vi "Tray_Search_ArrTrueIndex.vi"(6 "SearchStatus":bool=TRUE, 7 "Direction":u16=7, 10 "index":i32, 11 "Input_Arr":bool[][](array[boolean])) -> (1 "Status":bool, 2 "SearchTrueIndex":i32, 3 "indexTransXY":cluster{"Y":i32, "X":i32})   [LabVIEW 2015]
panel:
  out "indexTrans":i32
  out "Out XY 2":cluster{"Y":i32, "X":i32}
  out "Out XY":cluster{"Y":i32, "X":i32}
  out "Out PutArr":bool[][](array[boolean])
  # "X=(8-Y)-1\nY=(21-X)-1"
  # "4 6"
  # "8*21"
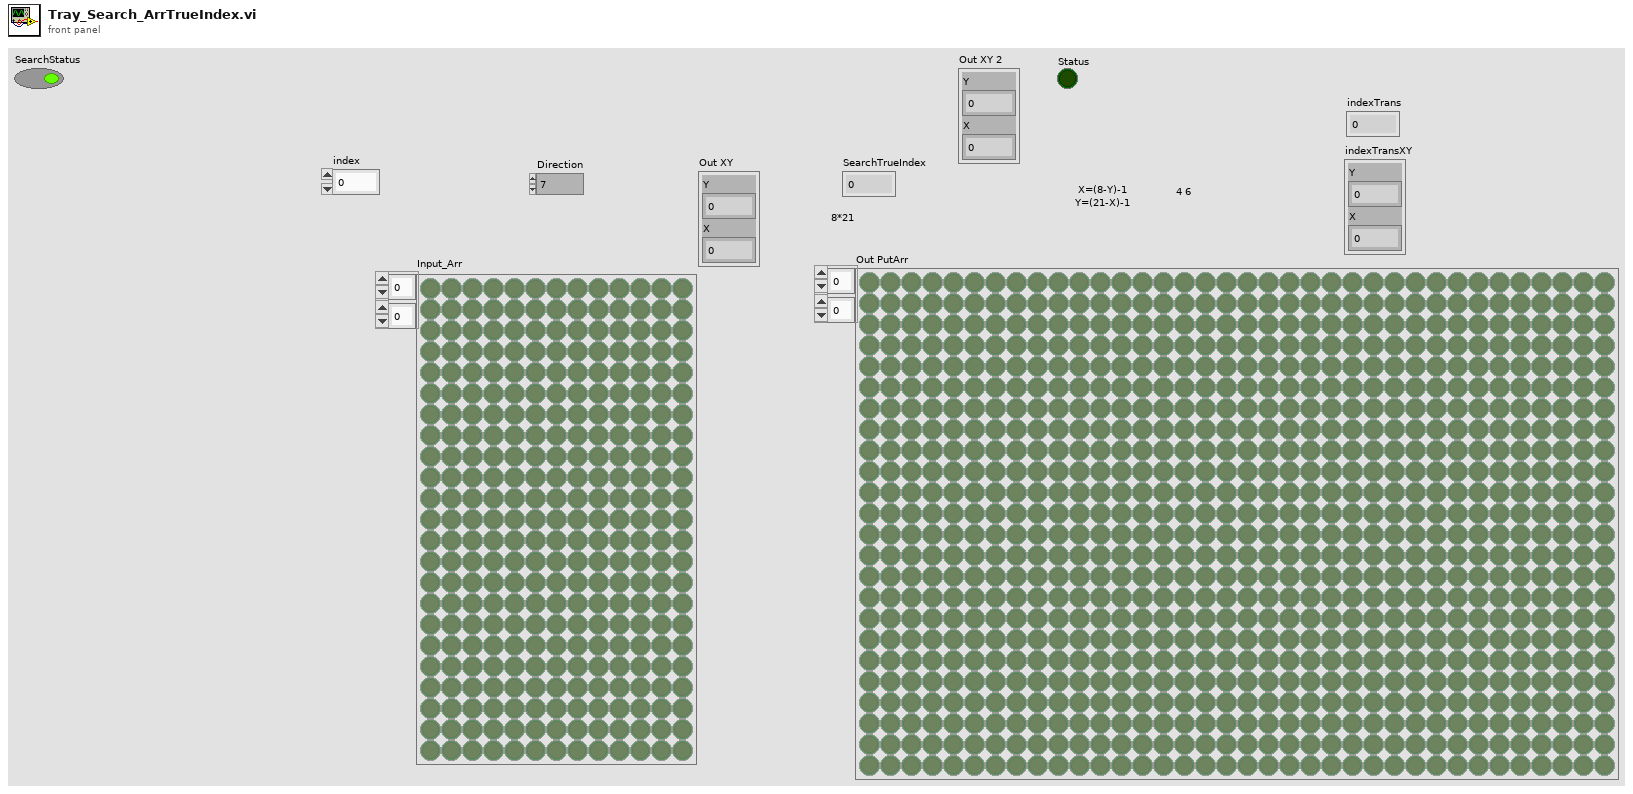
[diagram p1: front panel]
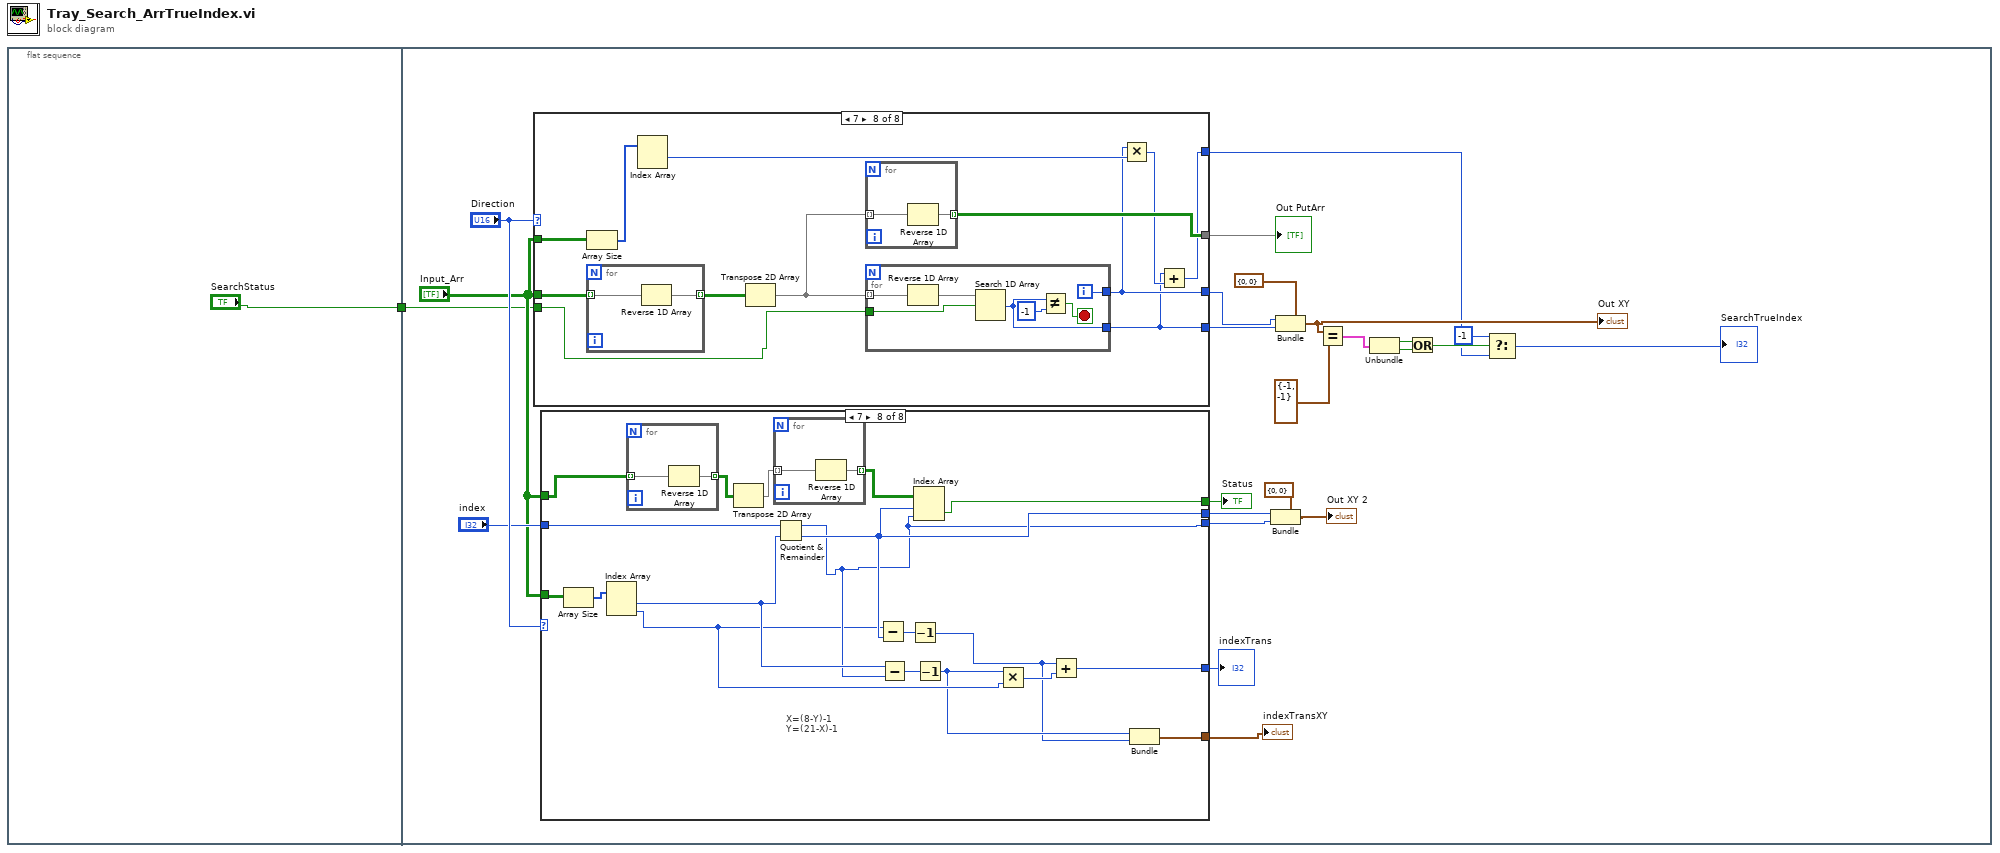
[diagram p0: block diagram]
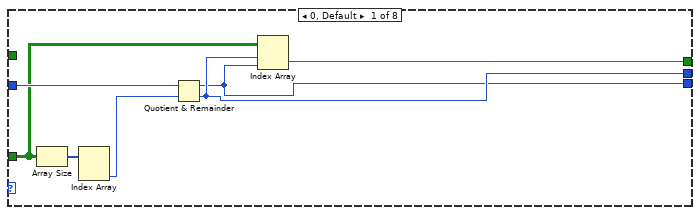
[diagram p2: hidden frame]
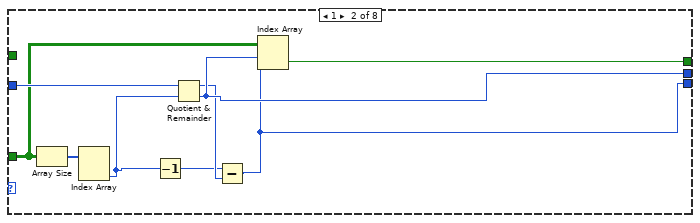
[diagram p3: hidden frame]
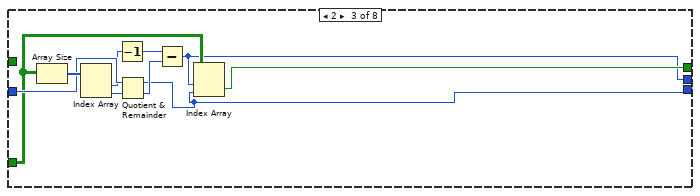
[diagram p4: hidden frame]
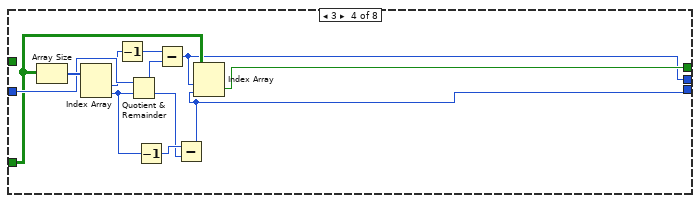
[diagram p5: hidden frame]
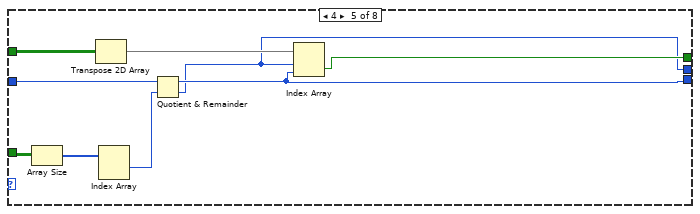
[diagram p6: hidden frame]
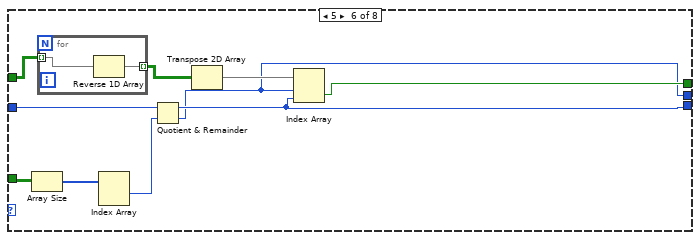
[diagram p7: hidden frame]
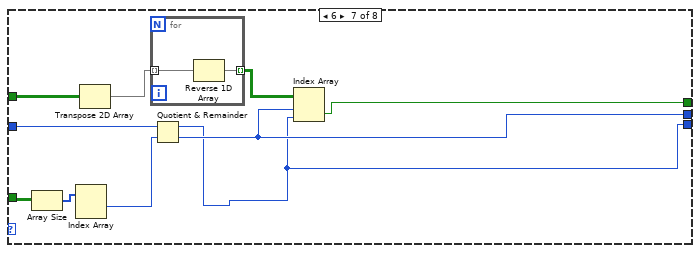
[diagram p8: hidden frame]
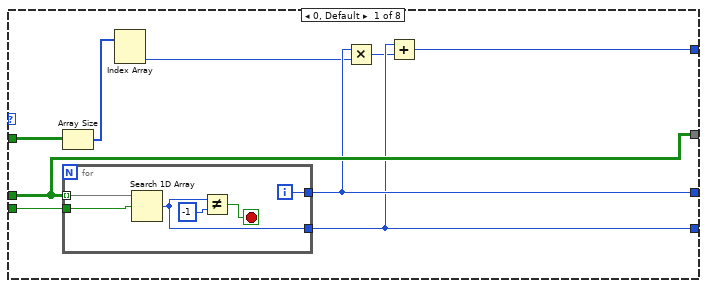
[diagram p9: hidden frame]
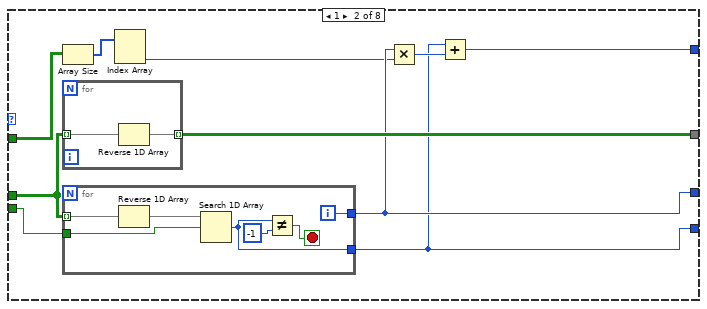
[diagram p10: hidden frame]
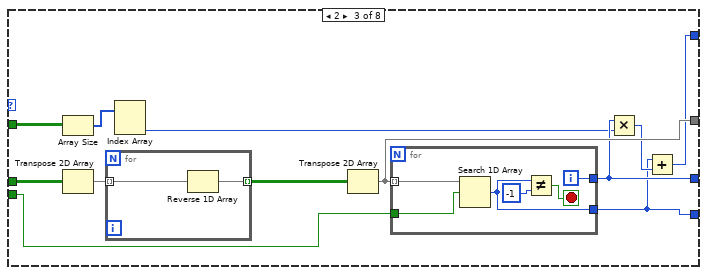
[diagram p11: hidden frame]
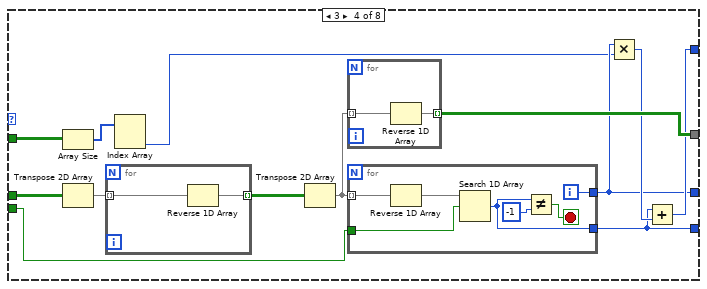
[diagram p12: hidden frame]
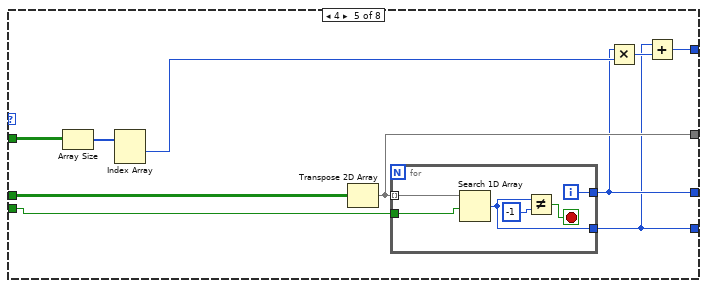
[diagram p13: hidden frame]
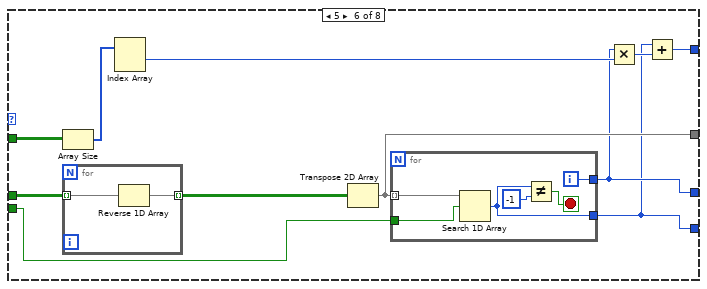
[diagram p14: hidden frame]
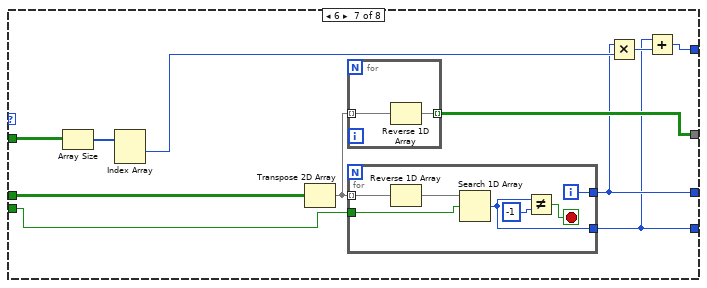
[diagram p15: hidden frame]
diagram:
  n1 = flat-sequence {
    tunnel: ["SearchStatus"] -> w1
    tunnel: w1 -> [w3]
    frame #0 {
    }
    frame #1 {
      n2 = case shown="7" "Direction" {
        tunnel: "Input_Arr" -> [w128 w144 w165 w186 w207 w224 w241 w262]
        tunnel: [w125 w139 w158 w177 w201 w217 w236 w256] -> w25
        tunnel: [w124 w138 w157 w176 w200 w216 w235 w255] -> w24
        tunnel: [w128 w143 w162 w182 w206 w222 w242 w263] -> w23
        tunnel: "Input_Arr" -> [w127 w140 w159 w179 w202 w218 w237 w257]
        tunnel: [w122 w137 w156 w178 w199 w215 w234 w254] -> w16
        tunnel: w3 -> [w120 w135 w154 w174 w198 w214 w233 w253]
        frame 0, Default {
          n3 = Array Size(array=w127) -> (size(s)=w126:i32[])
          n4 = for {
            tunnel: w128 -> [w134] mode=indexing
            tunnel: [w131] -> w125
            tunnel: [w130] -> w124
            tunnel: w120 -> [w129]
            i -> [w131]
            stop <- w132 stop-if-true
            n5 = Search 1D Array(1D array=w134, element=w129) -> (index of element=w130:i32)  [unwired: 1 in]
            n6 = Not Equal?(x=w130, y=-1) -> (x != y?=w132:bool)
          }
          n7 = Index Array(array=w126) -> (element #2=w121:i32)  [unwired: 2 in, 1 out]
          n8 = Multiply(x=w125, y=w121) -> (x*y=w123:i32)
          n9 = Add(x=w124, y=w123) -> (x+y=w122:i32)
        }
        frame 1 {
          n10 = Array Size(array=w140) -> (size(s)=w142:i32[])
          n11 = for {
            tunnel: w144 -> [w146] mode=indexing
            tunnel: [w145] -> w143 mode=indexing
            n12 = Reverse 1D Array(array=w146) -> (reversed array=w145:bool[])
          }
          n13 = for {
            tunnel: w144 -> [w153] mode=indexing
            tunnel: [w150] -> w139
            tunnel: [w149] -> w138
            tunnel: w135 -> [w147]
            i -> [w150]
            stop <- w151 stop-if-true
            n14 = Reverse 1D Array(array=w153) -> (reversed array=w148:bool[])
            n15 = Search 1D Array(1D array=w148, element=w147) -> (index of element=w149:i32)  [unwired: 1 in]
            n16 = Not Equal?(x=w149, y=-1) -> (x != y?=w151:bool)
          }
          n17 = Index Array(array=w142) -> (element #2=w136:i32)  [unwired: 2 in, 1 out]
          n18 = Multiply(x=w139, y=w136) -> (x*y=w141:i32)
          n19 = Add(x=w138, y=w141) -> (x+y=w137:i32)
        }
        frame 2 {
          n20 = Array Size(array=w159) -> (size(s)=w161:i32[])
          n21 = Transpose 2D Array(2D array=w165) -> (transposed array=w164:bool[][])
          n22 = for {
            tunnel: w164 -> [w167] mode=indexing
            tunnel: [w166] -> w163 mode=indexing
            n23 = Reverse 1D Array(array=w167) -> (reversed array=w166:bool[])
          }
          n24 = Index Array(array=w161) -> (element #2=w155:i32)  [unwired: 2 in, 1 out]
          n25 = Transpose 2D Array(2D array=w163) -> (transposed array=w162:bool[][])
          n26 = for {
            tunnel: w162 -> [w169] mode=indexing
            tunnel: [w171] -> w158
            tunnel: [w170] -> w157
            tunnel: w154 -> [w168]
            i -> [w171]
            stop <- w172 stop-if-true
            n27 = Search 1D Array(1D array=w169, element=w168) -> (index of element=w170:i32)  [unwired: 1 in]
            n28 = Not Equal?(x=w170, y=-1) -> (x != y?=w172:bool)
          }
          n29 = Multiply(x=w158, y=w155) -> (x*y=w160:i32)
          n30 = Add(x=w157, y=w160) -> (x+y=w156:i32)
        }
        frame 3 {
          n31 = Array Size(array=w179) -> (size(s)=w181:i32[])
          n32 = Transpose 2D Array(2D array=w186) -> (transposed array=w185:bool[][])
          n33 = for {
            tunnel: w185 -> [w190] mode=indexing
            tunnel: [w189] -> w184 mode=indexing
            n34 = Reverse 1D Array(array=w190) -> (reversed array=w189:bool[])
          }
          n35 = Index Array(array=w181) -> (element #2=w175:i32)  [unwired: 2 in, 1 out]
          n36 = Transpose 2D Array(2D array=w184) -> (transposed array=w183:bool[][])
          n37 = for {
            tunnel: w183 -> [w188] mode=indexing
            tunnel: [w187] -> w182 mode=indexing
            n38 = Reverse 1D Array(array=w188) -> (reversed array=w187:bool[])
          }
          n39 = for {
            tunnel: w183 -> [w193] mode=indexing
            tunnel: [w195] -> w177
            tunnel: [w194] -> w176
            tunnel: w174 -> [w191]
            i -> [w195]
            stop <- w196 stop-if-true
            n40 = Reverse 1D Array(array=w193) -> (reversed array=w192:bool[])
            n41 = Search 1D Array(1D array=w192, element=w191) -> (index of element=w194:i32)  [unwired: 1 in]
            n42 = Not Equal?(x=w194, y=-1) -> (x != y?=w196:bool)
          }
          n43 = Multiply(x=w177, y=w175) -> (x*y=w180:i32)
          n44 = Add(x=w176, y=w180) -> (x+y=w178:i32)
        }
        frame 4 {
          n45 = Array Size(array=w202) -> (size(s)=w205:i32[])
          n46 = Index Array(array=w205) -> (element #1=w204:i32)  [unwired: 2 in, 1 out]
          n47 = Transpose 2D Array(2D array=w207) -> (transposed array=w206:bool[][])
          n48 = for {
            tunnel: w206 -> [w211] mode=indexing
            tunnel: [w209] -> w200
            tunnel: [w210] -> w201
            tunnel: w198 -> [w208]
            i -> [w210]
            stop <- w212 stop-if-true
            n49 = Search 1D Array(1D array=w211, element=w208) -> (index of element=w209:i32)  [unwired: 1 in]
            n50 = Not Equal?(x=w209, y=-1) -> (x != y?=w212:bool)
          }
          n51 = Multiply(x=w201, y=w204) -> (x*y=w203:i32)
          n52 = Add(x=w200, y=w203) -> (x+y=w199:i32)
        }
        frame 5 {
          n53 = Array Size(array=w218) -> (size(s)=w221:i32[])
          n54 = for {
            tunnel: w224 -> [w226] mode=indexing
            tunnel: [w225] -> w223 mode=indexing
            n55 = Reverse 1D Array(array=w226) -> (reversed array=w225:bool[])
          }
          n56 = Index Array(array=w221) -> (element #1=w220:i32)  [unwired: 2 in, 1 out]
          n57 = Transpose 2D Array(2D array=w223) -> (transposed array=w222:bool[][])
          n58 = for {
            tunnel: w222 -> [w230] mode=indexing
            tunnel: [w229] -> w216
            tunnel: [w228] -> w217
            tunnel: w214 -> [w227]
            i -> [w228]
            stop <- w231 stop-if-true
            n59 = Search 1D Array(1D array=w230, element=w227) -> (index of element=w229:i32)  [unwired: 1 in]
            n60 = Not Equal?(x=w229, y=-1) -> (x != y?=w231:bool)
          }
          n61 = Multiply(x=w217, y=w220) -> (x*y=w219:i32)
          n62 = Add(x=w216, y=w219) -> (x+y=w215:i32)
        }
        frame 6 {
          n63 = Array Size(array=w237) -> (size(s)=w240:i32[])
          n64 = Index Array(array=w240) -> (element #1=w239:i32)  [unwired: 2 in, 1 out]
          n65 = Transpose 2D Array(2D array=w241) -> (transposed array=w243:bool[][])
          n66 = for {
            tunnel: w243 -> [w245] mode=indexing
            tunnel: [w244] -> w242 mode=indexing
            n67 = Reverse 1D Array(array=w245) -> (reversed array=w244:bool[])
          }
          n68 = for {
            tunnel: w243 -> [w250] mode=indexing
            tunnel: [w247] -> w235
            tunnel: [w248] -> w236
            tunnel: w233 -> [w246]
            i -> [w248]
            stop <- w251 stop-if-true
            n69 = Reverse 1D Array(array=w250) -> (reversed array=w249:bool[])
            n70 = Search 1D Array(1D array=w249, element=w246) -> (index of element=w247:i32)  [unwired: 1 in]
            n71 = Not Equal?(x=w247, y=-1) -> (x != y?=w251:bool)
          }
          n72 = Multiply(x=w236, y=w239) -> (x*y=w238:i32)
          n73 = Add(x=w235, y=w238) -> (x+y=w234:i32)
        }
        frame 7 {
          n74 = Array Size(array=w257) -> (size(s)=w260:i32[])
          n75 = for {
            tunnel: w262 -> [w266] mode=indexing
            tunnel: [w265] -> w261 mode=indexing
            n76 = Reverse 1D Array(array=w266) -> (reversed array=w265:bool[])
          }
          n77 = Index Array(array=w260) -> (element #1=w259:i32)  [unwired: 2 in, 1 out]
          n78 = Transpose 2D Array(2D array=w261) -> (transposed array=w264:bool[][])
          n79 = for {
            tunnel: w264 -> [w268] mode=indexing
            tunnel: [w267] -> w263 mode=indexing
            n80 = Reverse 1D Array(array=w268) -> (reversed array=w267:bool[])
          }
          n81 = for {
            tunnel: w264 -> [w273] mode=indexing
            tunnel: [w270] -> w255
            tunnel: [w271] -> w256
            tunnel: w253 -> [w269]
            i -> [w271]
            stop <- w274 stop-if-true
            n82 = Reverse 1D Array(array=w273) -> (reversed array=w272:bool[])
            n83 = Search 1D Array(1D array=w272, element=w269) -> (index of element=w270:i32)  [unwired: 1 in]
            n84 = Not Equal?(x=w270, y=-1) -> (x != y?=w274:bool)
          }
          n85 = Multiply(x=w256, y=w259) -> (x*y=w258:i32)
          n86 = Add(x=w255, y=w258) -> (x+y=w254:i32)
        }
      }
      "Out PutArr" <- w23
      n87 = case shown="7" "Direction" {
        tunnel: "index" -> [w32 w41 w51 w62 w70 w80 w92 w113]
        tunnel: "Input_Arr" -> [w30 w40 w50 w61 w71 w81 w93 w114]
        tunnel: [w29 w39 w46 w59 w64 w75 w90 w107] -> w10
        tunnel: [w28 w35 w43 w53 w65 w76 w85 w104] -> w9
        tunnel: [w27 w38 w49 w60 w68 w78 w91 w112] -> w8
        tunnel: "Input_Arr" -> [_ _ _ _ w67 w74 w89 w109]
        tunnel: [_ _ _ _ _ _ _ w100] -> w5
        tunnel: [_ _ _ _ _ _ _ w97] -> w4
        frame 0, Default {
          n88 = Array Size(array=w30) -> (size(s)=w33:i32[])
          n89 = Index Array(array=w33) -> (element #2=w31:i32)  [unwired: 2 in, 1 out]
          n90 = Quotient & Remainder(x=w32, y=w31) -> (x-y*floor(x/y)=w28:i32, floor(x/y)=w29:i32)
          n91 = Index Array(array=w30, index (row)=w29, index (col)=w28) -> (element=w27:bool)
        }
        frame 1 {
          n92 = Array Size(array=w40) -> (size(s)=w42:i32[])
          n93 = Index Array(array=w42) -> (element #2=w36:i32)  [unwired: 2 in, 1 out]
          n94 = Decrement(x=w36) -> (x-1=w34:i32)
          n95 = Quotient & Remainder(x=w41, y=w36) -> (x-y*floor(x/y)=w37:i32, floor(x/y)=w39:i32)
          n96 = Subtract(x=w34, y=w37) -> (x-y=w35:i32)
          n97 = Index Array(array=w40, index (row)=w39, index (col)=w35) -> (element=w38:bool)
        }
        frame 2 {
          n98 = Array Size(array=w50) -> (size(s)=w52:i32[])
          n99 = Index Array(array=w52) -> (element #1=w44:i32, element #2=w48:i32)  [unwired: 2 in]
          n100 = Decrement(x=w44) -> (x-1=w45:i32)
          n101 = Quotient & Remainder(x=w51, y=w48) -> (x-y*floor(x/y)=w43:i32, floor(x/y)=w47:i32)
          n102 = Subtract(x=w45, y=w47) -> (x-y=w46:i32)
          n103 = Index Array(array=w50, index (row)=w46, index (col)=w43) -> (element=w49:bool)
        }
        frame 3 {
          n104 = Array Size(array=w61) -> (size(s)=w63:i32[])
          n105 = Index Array(array=w63) -> (element #1=w57:i32, element #2=w56:i32)  [unwired: 2 in]
          n106 = Decrement(x=w57) -> (x-1=w58:i32)
          n107 = Quotient & Remainder(x=w62, y=w56) -> (floor(x/y)=w54:i32)  [unwired: 1 out]
          n108 = Decrement(x=w56) -> (x-1=w55:i32)
          n109 = Subtract(x=w58, y=w54) -> (x-y=w59:i32)
          n110 = Subtract(x=w55, y=w54) -> (x-y=w53:i32)
          n111 = Index Array(array=w61, index (row)=w59, index (col)=w53) -> (element=w60:bool)
        }
        frame 4 {
          n112 = Array Size(array=w71) -> (size(s)=w72:i32[])
          n113 = Transpose 2D Array(2D array=w67) -> (transposed array=w66:bool[][])
          n114 = Index Array(array=w72) -> (element #1=w69:i32)  [unwired: 2 in, 1 out]
          n115 = Quotient & Remainder(x=w70, y=w69) -> (x-y*floor(x/y)=w65:i32, floor(x/y)=w64:i32)
          n116 = Index Array(array=w66, index (row)=w64, index (col)=w65) -> (element=w68:bool)
        }
        frame 5 {
          n117 = Array Size(array=w81) -> (size(s)=w82:i32[])
          n118 = for {
            tunnel: [w84] -> w73 mode=indexing
            tunnel: w74 -> [w83] mode=indexing
            n119 = Reverse 1D Array(array=w83) -> (reversed array=w84:bool[])
          }
          n120 = Index Array(array=w82) -> (element #1=w79:i32)  [unwired: 2 in, 1 out]
          n121 = Quotient & Remainder(x=w80, y=w79) -> (x-y*floor(x/y)=w76:i32, floor(x/y)=w75:i32)
          n122 = Transpose 2D Array(2D array=w73) -> (transposed array=w77:bool[][])
          n123 = Index Array(array=w77, index (row)=w75, index (col)=w76) -> (element=w78:bool)
        }
        frame 6 {
          n124 = Array Size(array=w93) -> (size(s)=w94:i32[])
          n125 = Index Array(array=w94) -> (element #1=w86:i32)  [unwired: 2 in, 1 out]
          n126 = Transpose 2D Array(2D array=w89) -> (transposed array=w88:bool[][])
          n127 = for {
            tunnel: w88 -> [w96] mode=indexing
            tunnel: [w95] -> w87 mode=indexing
            n128 = Reverse 1D Array(array=w96) -> (reversed array=w95:bool[])
          }
          n129 = Quotient & Remainder(x=w92, y=w86) -> (x-y*floor(x/y)=w85:i32, floor(x/y)=w90:i32)
          n130 = Index Array(array=w87, index (row)=w90, index (col)=w85) -> (element=w91:bool)
        }
        frame 7 {
          # "X=(8-Y)-1\nY=(21-X)-1"
          n131 = Array Size(array=w114) -> (size(s)=w115:i32[])
          n132 = Index Array(array=w115) -> (element #1=w105:i32, element #2=w102:i32)  [unwired: 2 in]
          n133 = for {
            tunnel: w109 -> [w117] mode=indexing
            tunnel: [w116] -> w108 mode=indexing
            n134 = Reverse 1D Array(array=w117) -> (reversed array=w116:bool[])
          }
          n135 = Transpose 2D Array(2D array=w108) -> (transposed array=w111:bool[][])
          n136 = for {
            tunnel: w111 -> [w119] mode=indexing
            tunnel: [w118] -> w110 mode=indexing
            n137 = Reverse 1D Array(array=w119) -> (reversed array=w118:bool[])
          }
          n138 = Quotient & Remainder(x=w113, y=w105) -> (x-y*floor(x/y)=w104:i32, floor(x/y)=w107:i32)
          n139 = Subtract(x=w102, y=w107) -> (x-y=w106:i32)
          n140 = Subtract(x=w105, y=w104) -> (x-y=w103:i32)
          n141 = Decrement(x=w106) -> (x-1=w98:i32)
          n142 = Index Array(array=w110, index (row)=w107, index (col)=w104) -> (element=w112:bool)
          n143 = Decrement(x=w103) -> (x-1=w99:i32)
          n144 = Multiply(x=w99, y=w102) -> (x*y=w101:i32)
          n145 = Add(x=w98, y=w101) -> (x+y=w100:i32)
          n146 = Bundle(w99, w98) -> (w97:cluster{i32, i32})  [unwired: 1 in]
        }
      }
      "Status" <- w8
      "indexTrans" <- w5
      "indexTransXY" <- w4
      n147 = Bundle(cluster=cluster{"Y":i32, "X":i32} {"Y"=0, "X"=0} ("output cluster"), "Y"=w10, "X"=w9) -> (→"Out XY 2":cluster{"Y":i32, "X":i32})
      n148 = Bundle(cluster=cluster{"Y":i32, "X":i32} {"Y"=0, "X"=0} ("output cluster"), "Y"=w25, "X"=w24) -> (w21:cluster{"Y":i32, "X":i32})
      "Out XY" <- w21
      n149 = Equal?(x=w21, y=cluster{"Y":i32, "X":i32} {"Y"=-1, "X"=-1}) -> (x = y?=w20:cluster{"Y":bool, "X":bool})
      n150 = Unbundle(w20) -> ("Y"=w19:bool, "X"=w18:bool)
      n151 = Or(x=w19, y=w18) -> (x .or. y?=w17:bool)
      n152 = Select(t=-1, s=w17, f=w16) -> (s? t:f=→"SearchTrueIndex":i32)
    }
  }
